vi "Kazu_randstim_TMStrigger and cleaned_ver2.vi"() -> ()   [LabVIEW 2011]
uses:
  <vilib>/Analysis/NI_AALBase.lvlib
  <vilib>/DAQmx/create/channels.llb/DAQmx Create Channel (DO-Digital Output).vi
  <vilib>/DAQmx/write.llb/DAQmx Write (Digital Bool 1Line 1Point).vi
  <vilib>/Utility/file.llb/Read Delimited Spreadsheet (I64).vi
  <vilib>/Platform/TimedLoop/XDataNode/wakeup.ctl
  <vilib>/Platform/TimedLoop/XDataNode/XDNodeRunTimeDep.lvlib
  <vilib>/Platform/TimedLoop/XDataNode/nitl_modes.ctl
  <vilib>/Platform/TimedLoop/XDataNode/timing_clust.ctl
  <vilib>/platform/TimedLoop/XDataNode/XDataNode.xnode
  <vilib>/Analysis/baseanly.llb/A x Vector.vi
  <vilib>/Utility/file.llb/Write Delimited Spreadsheet (DBL).vi
  <vilib>/Platform/TimedLoop/scheduler/LVUserAPI/_suppVIs/Create_1kHz_TSource.vi
panel:
  in  "train length (ms)":i64=500
  out "TMS trigger send":bool
  in  "H duration (ms)":i32=10 min=5 max=15
  in  "DO duration (ms)":i32=500
  in  "nominal freq (Hz)":i32=40
  in  "percent for random":dbl=20.0
  out "Digital Waveform Graph":digitalwaveform(graph)={"t0"=timestamp(0 s since 1904-01-01), "dt"=0.001, "Y"={"transitions"=[], "data"=[[1], [1], [1], [1], [1], [1], [1], [1], [1], [1], [0], [0], [0], [0], [0], [0], [0], [0], [0], [0], [0], [0], [0], [0], [0], [0], [1], [1], [1], [1], [1], [1], [1], [1], [1], [1], [0], [0], [0], [0], [0], [0], [0], [0], [0], [0], [0], [0], [0], [0], [0], [1], [1], [1], [1], [1], [1], [1], [1], [1], [1], [0], [0], [0], [0], [0], [0], [0], [0], [0], [0], [0], [0], [0], [0], [1], [1], [1], [1], [1], [1], [1], [1], [1], [1], [0], [0], [0], [0], [0], [0], [0], [0], [0], [0], [0], [0], [0], [0], [0], [1], [1], [1], [1], [1], [1], [1], [1], [1], [1], [0], [0], [0], [0], [0], [0], [0], [0], [0], [0], [0], [0], [0], [0], [0], [0], [0], [0], [0], [0], [0], [0], [0], [0], [0], [0], [0], [0], [0], [0], [0], [0], [0], [0], [0], [0], [0], [0], [0], [0], [0], [0], [0], [0], [0], [0], [0], [0], [0], [0], [0], [0], [0], [0], [0], [0], [0], [0], [0], [0], [0], [0], [0], [0], [0], [0], [0], [0], [0], [0], [0], [0], [0], [0], [0], [0], [0], [0], [0], [0], [0], [0], [0], [0], [0], [0], [0], [0], [0], [0], [0], [0], [0], [0], [0], [0], [0], [0], [0], [0], [0], [0], [0], [0], [0], [0], [0], [0], [0], [0], [0], [0], [0], [0], [0], [0], [0], [0], [0], [0], [0], [0], [0], [0], [0], [0], [0], [0], [0], [0], [0], [0], [0], [0], [0], [0], [0], [0], [0], [0], [0], [0], [0], [0], [0], [0], [0], [0], [0], [0], [0], [0], [0], [0], [0], [0], [0], [0], [0], [0], [0], [0], [0], [0], [0], [0], [0], [0], [0], [0], [0], [0], [0], [0], [0], [0], [0], [0], [0], [0], [0], [0], [0], [0], [0], [0], [0], [0], [0], [0], [0], [0], [0], [0], [0], [0], [0], [0], [0], [0], [0], [0], [0], [0], [0], [0], [0], [0], [0], [0], [0], [0], [0], [0], [0], [0], [0], [0], [0], [0], [0], [0], [0], [0], [0], [0], [0], [0], [0], [0], [0], [0], [0], [0], [0], [0], [0], [0], [0], [0], [0], [0], [0], [0], [0], [0], [0], [0], [0], [0], [0], [0], [0], [0], [0], [0], [0], [0], [0], [0], [0], [0], [0], [0], [0], [0], [0], [0], [0], [0], [0], [0], [0], [0], [0], [0], [0], [0], [0], [0], [0], [0], [0], [0], [0], [0], [0], [0], [0], [0], [0], [0], [0], [0], [0], [0], [0], [0], [0], [0], [0], [0], [0], [0], [0], [0], [0], [0], [0], [0], [0], [0], [0], [0], [0], [0], [0], [0], [0], [0], [0], [0], [0], [0], [0], [0], [0], [0], [0], [0], [0], [0], [0], [0], [0], [0], [0], [0], [0], [0], [0], [0], [0], [0], [0], [0], [0], [0], [0], [0], [0], [0], [0], [0], [0], [0], [0], [0], [0], [0], [0], [0], [0], [0], [0], [0], [0], [0], [0], [0], [0], [0], [0], [0], [0], [0], [0], [0], [0], [0], [0], [0], [0], [0], [0], [0], [0], [0], [0], [0]]}}
  in  "Trial No":u16(ring)=1 items=["N/A", "Trial 1", "Trial 2", "Trial 3", "Trial 4", "Trial 5", "Trial 6", "Trial 7", "Trial 8", "Trial 9", "Trial 10", "Trial 11", "Trial 12", "Trial 13", "Trial 14", "Trial 15", "Trial 16", "Trial 17", "Trial 18", "Trial 19", "Trial 20", "Trial 21", "Trial 22", "Trial 23", "Trial 24", "Trial 25", "Trial 26", "Trial 27", "Trial 28", "Trial 29", "Trial 30", "Trial 31", "Trial 32", "Trial 33", "Trial 34", "Trial 35", "Trial 36", "Trial 37", "Trial 38", "Trial 39", "Trial 40", "Trial 41", "Trial 42", "Trial 43", "Trial 44", "Trial 45", "Trial 46", "Trial 47", "Trial 48", "Trial 49", "Trial 50", "Trial 51", "Trial 52", "Trial 53", "Trial 54", "Trial 55", "Trial 56", "Trial 57", "Trial 58", "Trial 59", "Trial 60", "Trial 61", "Trial 62", "Trial 63", "Trial 64", "Trial 65", "Trial 66", "Trial 67", "Trial 68", "Trial 69", "Trial 70", "Trial 71", "Trial 72", "Trial 73", "Trial 74", "Trial 75", "Trial 76", "Trial 77", "Trial 78", "Trial 79", "Trial 80", "Trial 81", "Trial 82", "Trial 83", "Trial 84", "Trial 85", "Trial 86", "Trial 87", "Trial 88", "Trial 89", "Trial 90", "Trial 91", "Trial 92", "Trial 93", "Trial 94", "Trial 95", "Trial 96", "Trial 97", "Trial 98", "Trial 99", "Trial 100", "Trial 101", "Trial 102", "Trial 103", "Trial 104", "Trial 105", "Trial 106", "Trial 107", "Trial 108", "Trial 109", "Trial 110", "Trial 111", "Trial 112", "Trial 113", "Trial 114", "Trial 115", "Trial 116", "Trial 117", "Trial 118", "Trial 119", "Trial 120", "Trial 121", "Trial 122", "Trial 123", "Trial 124", "Trial 125", "Trial 126", "Trial 127", "Trial 128", "Trial 129", "Trial 130", "Trial 131", "Trial 132", "Trial 133", "Trial 134", "Trial 135", "Trial 136", "Trial 137", "Trial 138", "Trial 139", "Trial 140", "Trial 141", "Trial 142", "Trial 143", "Trial 144", "Trial 145", "Trial 146", "Trial 147", "Trial 148", "Trial 149", "Trial 150", "Trial 151", "Trial 152", "Trial 153", "Trial 154", "Trial 155", "Trial 156", "Trial 157", "Trial 158", "Trial 159", "Trial 160", "Trial 161", "Trial 162", "Trial 163", "Trial 164", "Trial 165", "Trial 166", "Trial 167", "Trial 168", "Trial 169", "Trial 170", "Trial 171", "Trial 172", "Trial 173", "Trial 174", "Trial 175", "Trial 176", "Trial 177", "Trial 178", "Trial 179", "Trial 180", "Trial 181", "Trial 182", "Trial 183", "Trial 184", "Trial 185", "Trial 186", "Trial 187", "Trial 188", "Trial 189", "Trial 190"]
  out "start":bool
  in  "RECORD":bool
  in  "BNC port for EMG":tag="Dev1/port0/line4" caption="BNC port for EMG and EMG"
  out "sucsess":bool
  out "TMS type":i64=3
  in  "sequence file path_TMS Order":path=path "C:/Users/marco2013/Documents/Kazu/EEG-TMS/rand_stim_study/rand_stim_taskorder/sub9/randStim_TMSOrder_sub9.txt"
  out "x-y":dbl=10.0
  out "checkTime":dbl=16261.0
  in  "MVC clear":bool
  out "MVC value":dbl=23.092750263611816
  in  "MVC recording":bool
  in  "total time":u32=9000
  out "timer":u32=16261
  out "end":bool
  out "go":bool
  out "ready":bool
  out "cue":bool
  out "%MVC":dbl(slide)=-0.42778761105628194 scale=0.0..60.0
  in  "BNC port for TMS":tag="Dev1/port0/line1"
  out "condtion":i64=1
  in  "sequence file path_TASK Order":path=path "C:/Users/marco2013/Documents/Kazu/EEG-TMS/rand_stim_study/rand_stim_taskorder/sub9/randStim_TaskOrder_sub9.txt"
  out "Force":dbl=-0.09878792467989823
  in  "Block":u16(ring)=1 items=["N/A", "Block 1", "Block 2", "Block 3", ""]
  in  "string":string="C:\\Users\\marco2013\\Documents\\Kazu\\EEG-TMS\\rand_stim_study\\"
  out "path":path=path "C:/Users/marco2013/Documents/Kazu/EEG-TMS/rand_stim_study/FT0101190.txt"
  in  "Subject":u16(ring)=9 items=["N/A", "Sub 1", "Sub 2", "Sub 3", "Sub 4", "Sub 5", "Sub 6", "Sub 7", "Sub 8", "Sub 9", "Sub 10", "Sub 11", "Sub 12", "Sub 13", "Sub 14", "Sub 15"]
  in  "number of samples":i32=10
  in  "device name":tag="Dev1"
  in  "Sampling rate":dbl=1000.0
  out "Array":dbl[][](array[numeric])=[[0.0, 0.0, 0.0, 0.0, 0.0, 0.0], [0.0, 0.0, 0.0, 0.0, 0.0, 0.0], [0.0, 0.0, 0.0, 0.0, 0.0, 0.0], [0.0, 0.0, 0.0, 0.0, 0.0, 0.0], [0.2289245236771016, -0.066272275562497, 0.09878792467989823, 0.001145934848439327, -0.0024626830830202645, -0.003738509500700172]]
  in  "stop":bool=TRUE
  in  "Bias All":bool
  in  "Enable Transducer 2":bool[](array[boolean])=[TRUE, TRUE, TRUE, TRUE, TRUE]
  in  "Calibration Files":path[](array[path])=[path "C:/Users/marco2013/Documents/Kazu/bigbox/FT6124.cal", path "C:/Users/marco2013/Documents/Kazu/bigbox/FT6561.cal", path "C:/Users/marco2013/Documents/Kazu/bigbox/FT4554.cal", path "C:/Users/marco2013/Documents/Kazu/bigbox/FT16536.cal", path "C:/Users/marco2013/Documents/Kazu/bigbox/FT14450.cal"]
  # "1: catch\n2: 20Hz stim\n3: 50Hz stim"
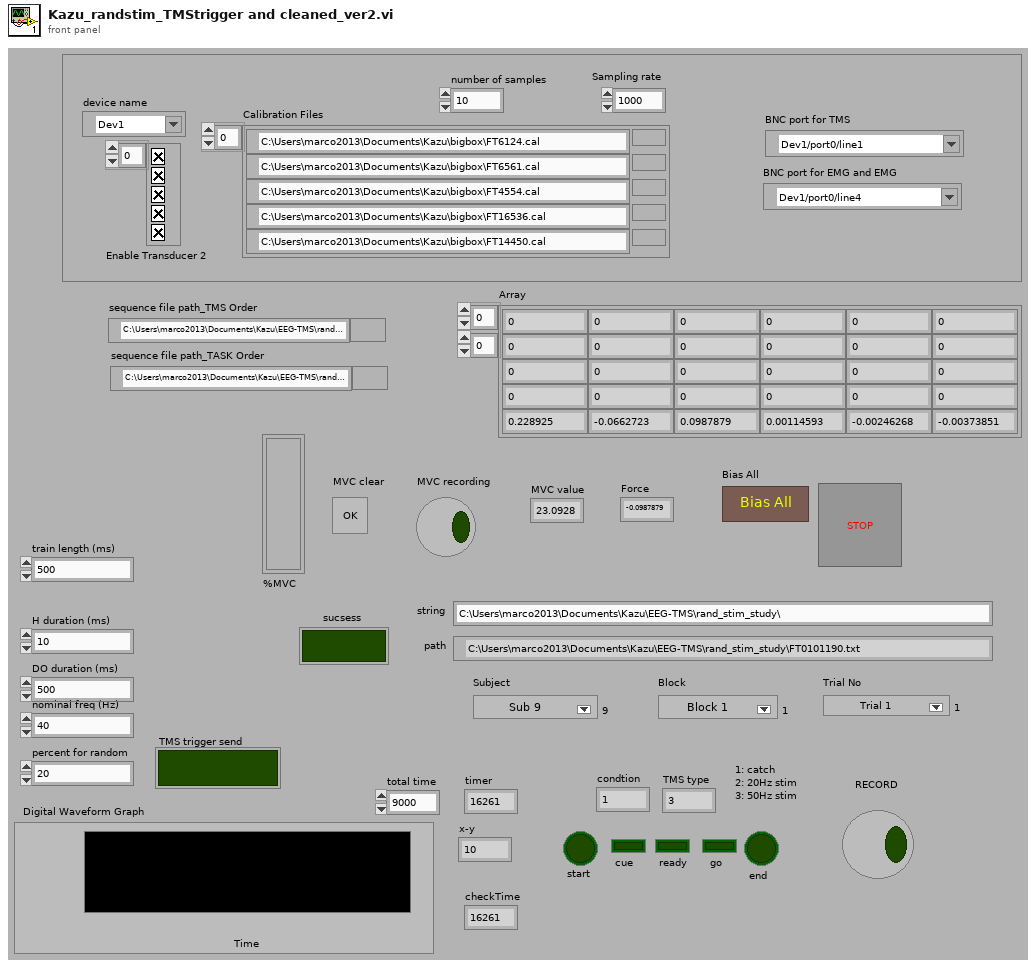
[diagram p1: front panel]
types:
  T1 = enum16{"open", "replace", "create", "open or create", "replace or create", "replace or create with confirmation"}
  T2 = enum16{"open", "open or create", "create or replace", "create", "open (read-only)"}
  T3 = typedef "XDNodeRunTimeDep.lvlib/timing_clust.ctl" = cluster{"Expected End [f-1]":u64, "Actual End [f-1]":u64, "Finished Late? [f-1]":bool, "Expected End [i-1]":u64, "Actual End [i-1]":u64, "Finished Late? [i-1]":bool, "Expected Start [i]":u64, "Actual Start [i]":u64, "Expected Start [f]":u64, "Actual Start [f]":u64, "Source Name":string, "Structure Name":string, "Period":i64, "Deadline":i64, "Offset":i64, "Start":i64, "Priority":i32, "Timeout":i32, "Mode":T4, "Wakeup Reason":T5, "Error":errorcluster, "Source Type":string, "Secondary Source Type":string, "Global End Time":u64, "Global Start Time":u64, "Frame Duration":u64, "Iteration Duration":u64, "Assigned CPU":i32, "I/O Scan Engine Mode":u32}
  T4 = typedef "XDNodeRunTimeDep.lvlib/nitl_modes.ctl" = enum32{"No Change", "Process missed periods, maintain original phase", "Discard missed periods, maintain original phase", "Process missed periods, ignore original phase", "Discard missed periods, ignore original phase"}
  T5 = typedef "XDNodeRunTimeDep.lvlib/wakeup.ctl" = enum32{"Normal", "Aborted", "Asynchronous wakeup", "Timing source error", "Timed loop error", "Timeout"}
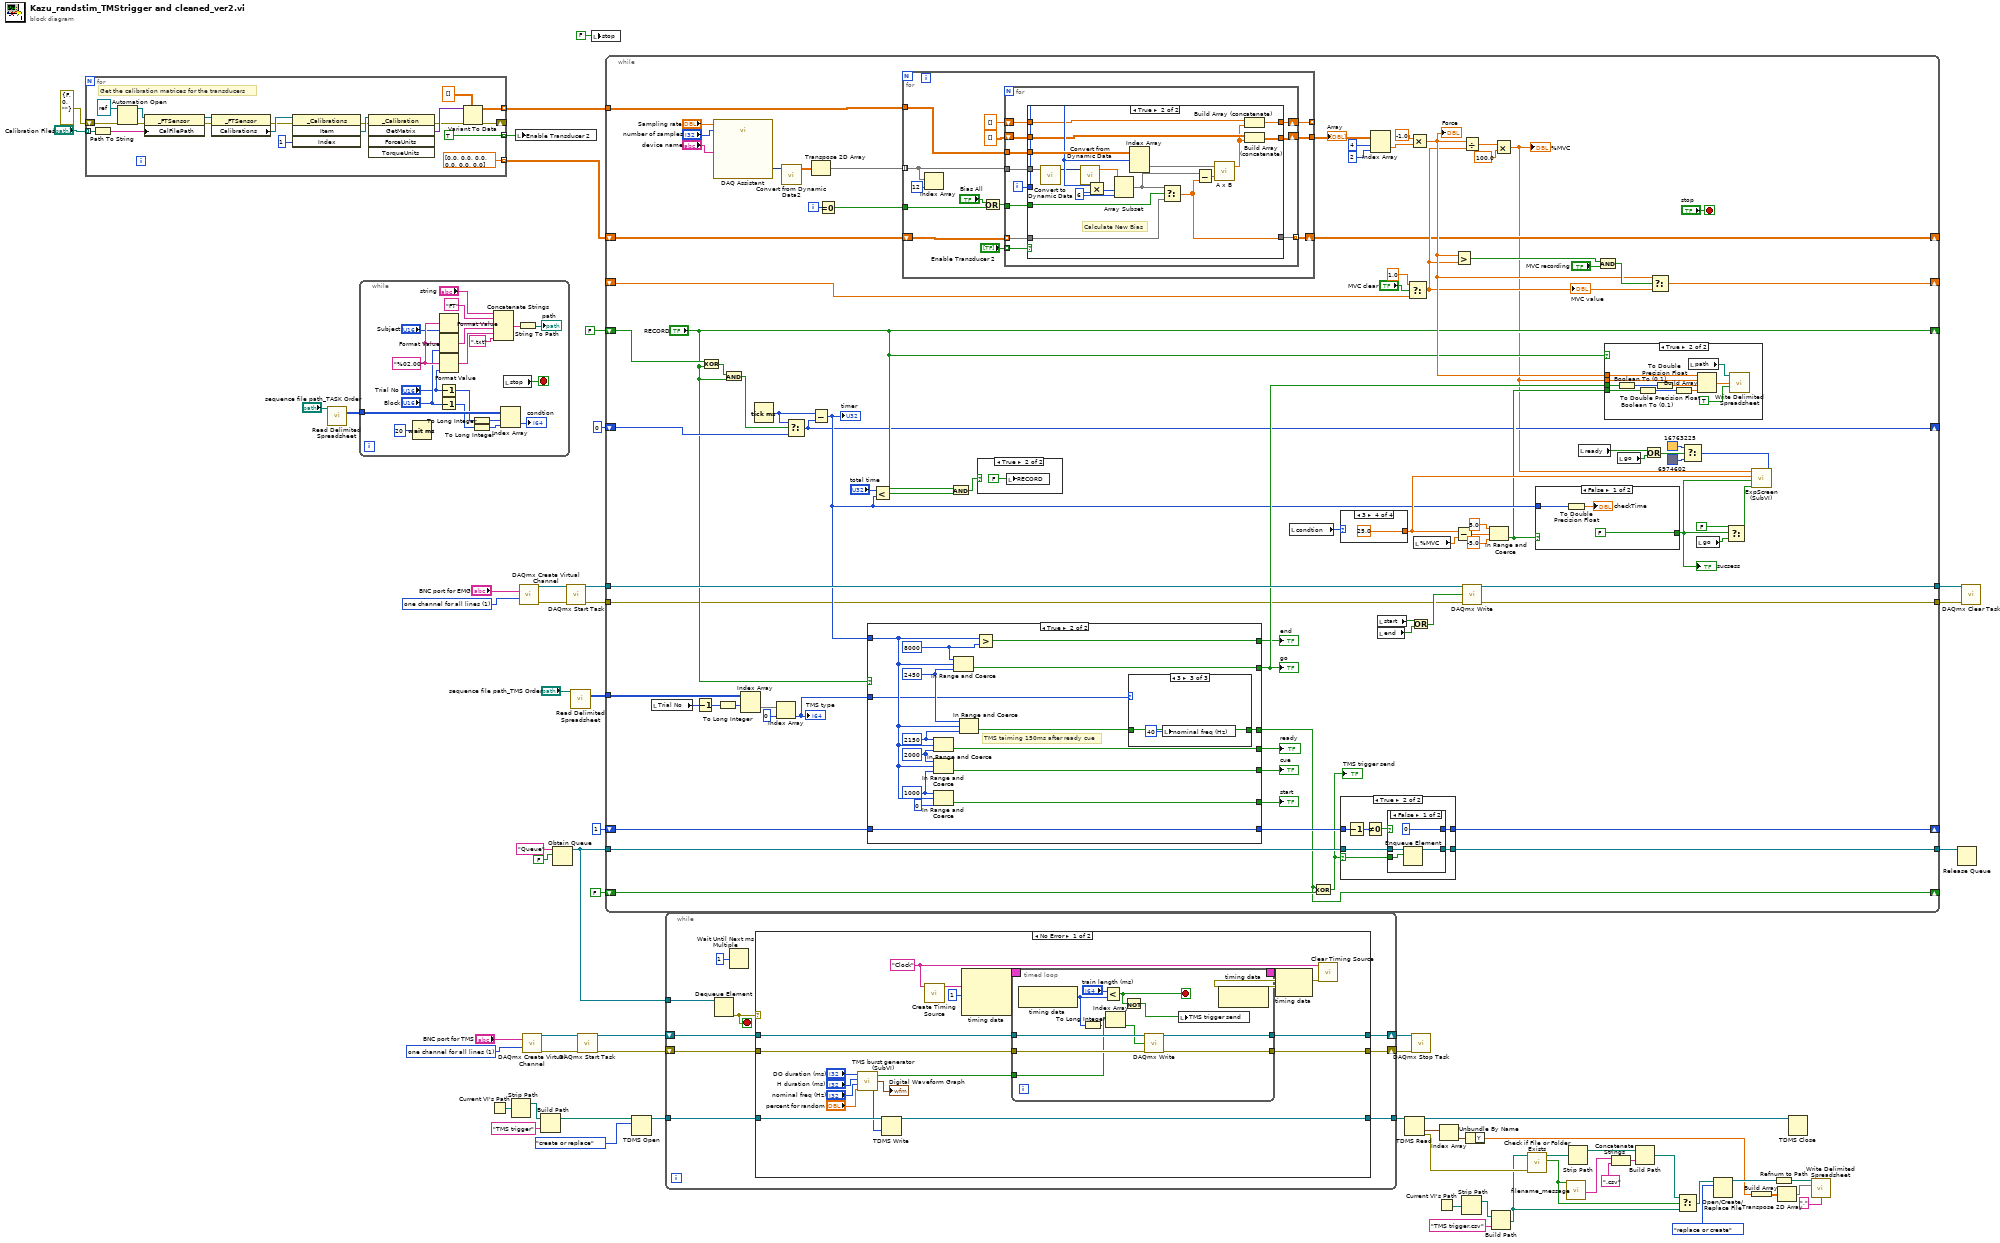
[diagram p0: block diagram]
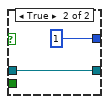
[diagram p4: hidden frame]
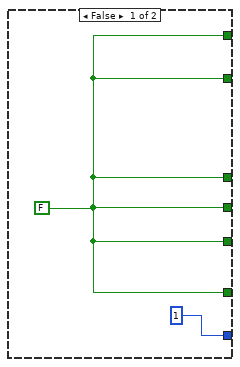
[diagram p6: hidden frame]
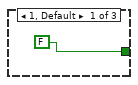
[diagram p7: hidden frame]
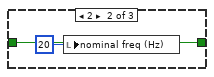
[diagram p8: hidden frame]
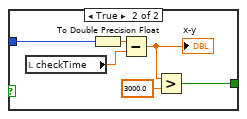
[diagram p9: hidden frame]
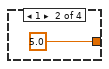
[diagram p11: hidden frame]
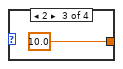
[diagram p12: hidden frame]
diagram:
  w51 = 1 items=["one channel for each line", "one channel for all lines"] ("line grouping")
  w55 = 1 items=["one channel for each line", "one channel for all lines"] ("line grouping")
  n1 = for {
    tunnel: "Calibration Files" -> [w81] mode=indexing
    shift-right: [w72] -> _
    shift-left: errorcluster {"status"=FALSE, "code"=0, "source"=""} ("error out") -> [w69]
    tunnel: [sgl[] [0.0, 0.0, 0.0, 0.0, 0.0, 0.0]] -> w60 mode=indexing
    tunnel: [TRUE] -> w62 mode=indexing
    tunnel: [w65] -> w61 mode=indexing
    # "Get the calibration matrices for the transducers"
    n2 = Path To String(path=w81) -> (string=w80:string)
    n3 = Automation Open(error in (no error)=w69, Automation Refnum=refnum<k7> refnum ("ATIDAQFT._FTSensor")) -> (Automation Refnum=w70:refnum<k7>, error out=w68:errorcluster)  [unwired: 1 in, 1 out]
    n4 = property on="Property Node" class="_FTSensor"(reference=w70, error in=w68, "CalFilePath"=w80) -> (reference out=w82:refnum<k7>, error out=w76:errorcluster)
    n5 = property class="_FTSensor"(reference=w82, error in=w76) -> (error out=w75:errorcluster, "Calibrations"=w84:refnum<k7>)  [unwired: 1 out]
    n6 = invoke class="_Calibrations" method="Item"(reference=w84, error in=w75, "Index"=1) -> (error out=w74:errorcluster, "Item"=w79:refnum<k7>)  [unwired: 1 in, 2 out]
    n7 = invoke class="_Calibration" method="GetMatrix"(reference=w79, error in=w74) -> (error out=w73:errorcluster, "GetMatrix"=w78:variant)  [unwired: 3 in, 3 out]
    n8 = Variant To Data(error in=w73, type=sgl[][] [], Variant=w78) -> (data=w65:sgl[][], error out=w72:errorcluster)
  }
  n9 = call-poly <vilib>:"Read Delimited Spreadsheet.vi"("file path (dialog if empty)"="sequence file path_TASK Order") -> ("all rows"=w56:i64[][])  [unwired: 9 in, 5 out]
  n10 = while {
    tunnel: w56 -> [w92]
    stop <- w104 stop-if-true
    w103 = "%02.00" ("string (\"\")")
    n11 = Wait (ms)(milliseconds to wait=u32 20) -> ()  [unwired: 1 out]
    n12 = Format Value(format string=w103, value (0)="Subject") -> (output string=w96:string)  [unwired: 1 out]
    n13 = Format Value(format string=w103, value (0)="Block") -> (output string=w102:string)  [unwired: 1 out]
    n14 = Format Value(format string=w103, value (0)="Trial No") -> (output string=w101:string)  [unwired: 1 out]
    n15 = Decrement(x="Trial No") -> (x-1=w90:u16)
    n16 = Decrement(x="Block") -> (x-1=w89:u16)
    n17 = To Long Integer(number=w90) -> (32bit integer=w86:i32)
    n18 = To Long Integer(number=w89) -> (32bit integer=w85:i32)
    n19 = Concatenate Strings("string", "FT", w96, w102, w101, ".txt") -> (w94:string)
    n20 = Index Array(array=w92, index (row)=w86, index (col)=w85) -> (element=→"condtion":i64)
    n21 = local read "stop"() -> (w104:bool)
    n22 = String To Path(string=w94) -> (path=→"path":path)
  }
  n23 = Current VI's Path() -> (path=w28:path)
  n24 = Strip Path(path=w28) -> (stripped path=w27:path)  [unwired: 1 out]
  n25 = local write "Enable Transducer 2"(w62) -> ()
  n26 = call-poly <vilib>:"DAQmx Create Virtual Channel.vi"("lines"="BNC port for EMG", "line grouping"=w51) -> ("task out"=w48:refnum<k21>, "error out"=w49:errorcluster)  [unwired: 3 in, 9 out]
  n27 = call-poly <vilib>:"DAQmx Create Virtual Channel.vi"("lines"="BNC port for TMS", "line grouping"=w55) -> ("task out"=w38:refnum<k21>, "error out"=w37:errorcluster)  [unwired: 3 in, 9 out]
  n28 = Build Path(base path=w27, name or relative path="TMS trigger") -> (appended path=w26:path)
  n29 = Obtain Queue(name (unnamed)="Queue", element data type=FALSE) -> (queue out=w33:refnum<queue>)  [unwired: 3 in, 2 out]
  n30 = call <vilib>:"DAQmx Start Task.vi"("task/channels in"=w48, "error in"=w49) -> ("task out"=w46:refnum<k21>, "error out"=w44:errorcluster)  [unwired: 12 out]
  n31 = call-poly <vilib>:"Read Delimited Spreadsheet.vi"("file path (dialog if empty)"="sequence file path_TMS Order") -> ("all rows"=w52:i64[][])  [unwired: 9 in, 5 out]
  n32 = call <vilib>:"DAQmx Start Task.vi"("task/channels in"=w38, "error in"=w37) -> ("task out"=w42:refnum<k21>, "error out"=w40:errorcluster)  [unwired: 12 in]
  n33 = local write "stop"(FALSE ("stop")) -> ()
  n34 = while {
    tunnel: w61 -> [w187]
    shift-right: [w159] -> _
    shift-left: w60 -> [w188]
    shift-right: ["RECORD"] -> _
    shift-left: FALSE -> [w176]
    shift-right: [w120] -> _
    shift-left: u32 0 ("millisecond timer value") -> [w136]
    shift-right: [w164] -> _
    shift-left: _ -> [w161]
    tunnel: w52 -> [w151]
    tunnel: [w149] -> w47
    tunnel: w46 -> [w148]
    tunnel: w44 -> [w116]
    tunnel: [w115] -> w43
    tunnel: w33 -> [w111]
    shift-right: [w108] -> _
    shift-left: FALSE ("RECORD") -> [w114]
    tunnel: [w109] -> w34
    shift-right: [w110] -> _
    shift-left: 1 -> [w113]
    i -> [w181]
    stop <- "stop" stop-if-true
    n35 = local read "Trial No"() -> (w119:u16)
    n36 = Decrement(x=w119) -> (x-1=w118:u16)
    n37 = Exclusive Or(1:"RECORD", 2:w176) -> (0:w135:bool)
    n38 = call "DAQ Assistant"("rate"="Sampling rate", "number of samples"="number of samples", "device name"="device name") -> ("data"=w184:dynamicdata)  [unwired: 3 in, 13 out]
    n39 = To Long Integer(number=w118) -> (32bit integer=w117:i32)
    n40 = And(x=w135, y="RECORD") -> (x .and. y?=w138:bool)
    n41 = Index Array(array=w151, index (row)=w117) -> (element=w152:i64[])  [unwired: 1 in]
    n42 = Tick Count (ms)() -> (millisecond timer value=w137:u32)
    n43 = Index Array(array=w152, index=0) -> (element=w150:i64)
    "TMS type" <- w150
    n44 = call "Convert from Dynamic Data2"("Dynamic Data Type"=w184) -> ("Array"=w183:dbl[][])  [unwired: 3 out]
    n45 = Select(t=w137, s=w138, f=w136) -> (s? t:f=w120:u32)
    n46 = Transpose 2D Array(2D array=w183) -> (transposed array=w182:dbl[][])
    n47 = Subtract(x=w137, y=w120) -> (x-y=w130:u32)
    "timer" <- w130
    n48 = Equal To 0?(x=w181) -> (x = 0?=w185:bool)
    n49 = case shown="True" "RECORD" {
      tunnel: [w206 w222] -> w139
      tunnel: [w206 w221] -> w145
      tunnel: [w206 w220] -> w141
      tunnel: [w206 w219] -> w140
      tunnel: [w206 w218] -> w146
      tunnel: w130 -> [_ w217]
      tunnel: [w206 w208] -> w108
      tunnel: w150 -> [_ w210]
      tunnel: [1 w216] -> w112
      tunnel: w113 -> [_ w216]
      frame False {
        w206 = FALSE ("RECORD")
      }
      frame True {
        w211 = u32 2450 ("upper limit")
        w212 = u32 8000 ("upper limit")
        w207 = u32 2150 ("upper limit")
        w213 = u32 2000 ("upper limit")
        w214 = u32 1000 ("upper limit")
        # "TMS taiming 150ms after ready cue"
        n50 = In Range and Coerce(upper limit=w207, x=w217, lower limit=w213) -> (In Range?=w219:bool)  [unwired: 1 out]
        n51 = In Range and Coerce(upper limit=w213, x=w217, lower limit=w214) -> (In Range?=w221:bool)  [unwired: 1 out]
        n52 = In Range and Coerce(upper limit=w214, x=w217, lower limit=u32 0) -> (In Range?=w222:bool)  [unwired: 1 out]
        n53 = In Range and Coerce(upper limit=w212, x=w217, lower limit=w211) -> (In Range?=w218:bool)  [unwired: 1 out]
        n54 = In Range and Coerce(upper limit=w211, x=w217, lower limit=w207) -> (In Range?=w209:bool)  [unwired: 1 out]
        n55 = Greater?(x=w217, y=w212) -> (0:w220:bool)
        n56 = case shown="3" w210 {
          tunnel: w209 -> [_ w224 w226]
          tunnel: [FALSE w224 w226] -> w208
          frame 1, Default {
          }
          frame 2 {
            n57 = local write "nominal freq (Hz)"(20 ("x")) -> ()
          }
          frame 3 {
            n58 = local write "nominal freq (Hz)"(40 ("x")) -> ()
          }
        }
      }
    }
    "ready" <- w140
    "cue" <- w145
    "go" <- w146
    "end" <- w141
    "start" <- w139
    n59 = Less?(x="total time", y=w130) -> (x < y?=w170:bool)
    n60 = for {
      tunnel: w182 -> [w252] mode=indexing
      tunnel: w187 -> [w263]
      shift-right: [w261] -> w159
      shift-left: w188 -> [w255]
      tunnel: w185 -> [w256]
      tunnel: [w254] -> w169
      tunnel: [w251] -> _ mode=indexing
      n61 = Index Array(array=w252, index=12) -> ()  [unwired: 1 out]
      n62 = Or(x="Bias All", y=w256) -> (x .or. y?=w257:bool)
      n63 = for {
        tunnel: w263 -> [w271]
        tunnel: w252 -> [w274]
        tunnel: w255 -> [w273] mode=indexing
        tunnel: [w272] -> w261 mode=indexing
        shift-right: [w264] -> w251
        shift-left: dbl[] [] -> [w269]
        tunnel: "Enable Transducer 2" -> [w268] mode=indexing
        shift-right: [w266] -> w254
        shift-left: sgl[][] [] -> [w267]
        tunnel: w257 -> [w265]
        i -> [w270]
        n64 = case shown="True" w268 {
          tunnel: w274 -> [_ w293]
          tunnel: w273 -> [w277 w279]
          tunnel: [w277 w280] -> w272
          tunnel: w271 -> [_ w291]
          tunnel: w270 -> [_ w289]
          tunnel: w269 -> [w276 w285]
          tunnel: [w276 w283] -> w264
          tunnel: w267 -> [w275 w288]
          tunnel: [w275 w287] -> w266
          tunnel: w265 -> [_ w281]
          frame False {
          }
          frame True {
            w294 = 6
            # "Calculate New Bias"
            n65 = call "Convert to Dynamic Data"("Array"=w293) -> ("Dynamic Data Type"=w282:dynamicdata)  [unwired: 3 out]
            n66 = call "Convert from Dynamic Data"("Dynamic Data Type"=w282) -> ("Array"=w286:dbl[])  [unwired: 3 out]
            n67 = Multiply(x=w289, y=w294) -> (x*y=w295:i32)
            n68 = Array Subset(array=w286, index=w295, length=w294) -> (w278:dbl[])
            n69 = Index Array(array=w291, index (dim 0)=w289) -> (element=w290:sgl[][])  [unwired: 2 in]
            n70 = Select(t=w278, s=w281, f=w279) -> (s? t:f=w280:dbl[])
            n71 = Subtract(x=w278, y=w280) -> (x-y=w292:dbl[])
            n72 = call-poly <vilib>:"A x B.vi"("Vector"=w292, "A"=w290) -> ("A x Vector"=w284:dbl[])  [unwired: 1 out]
            n73 = Build Array (concatenate)(w285, w284) -> (w283:dbl[])
            n74 = Build Array (concatenate)(w288, w284) -> (w287:dbl[][])
          }
        }
      }
    }
    "Array" <- w169
    n75 = And(x="RECORD", y=w170) -> (x .and. y?=w147:bool)
    n76 = case shown="True" w147 {
      frame False {
      }
      frame True {
        n77 = local write "RECORD"(FALSE ("RECORD")) -> ()
      }
    }
    n78 = local read "condtion"() -> (w158:i64)
    n79 = Exclusive Or(1:w114, 2:w108) -> (0:w107:bool)
    "TMS trigger send" <- w107
    n80 = case shown="3" w158 {
      tunnel: [_ 5.0 10.0 25.0] -> w157
      frame 0, Default {
      }
      frame 1 {
      }
      frame 2 {
      }
      frame 3 {
      }
    }
    n81 = case shown="True" w107 {
      selector: w107 -> [_ w194]
      tunnel: w112 -> [w190 w197]
      tunnel: w111 -> [w189 w193]
      tunnel: [w190 w192] -> w110
      tunnel: [w189 w191] -> w109
      frame False {
      }
      frame True {
        n82 = Decrement(x=w197) -> (x-1=w196:i32)
        n83 = Not Equal To 0?(x=w196) -> (x != 0?=w195:bool)
        n84 = case shown="False" w195 {
          tunnel: [0 1] -> w192
          tunnel: w194 -> [w201 _]
          tunnel: w193 -> [w200 w202]
          tunnel: [w198 w202] -> w191
          frame False {
            n85 = Enqueue Element(queue=w200, element=w201) -> (queue out=w198:refnum<queue>)  [unwired: 2 in, 2 out]
          }
          frame True {
          }
        }
      }
    }
    n86 = Index Array(array=w169, index (row)=4, index (col)=2 ("disabled index (col)")) -> (element=w175:dbl)
    n87 = local read "start"() -> (w144:bool)
    n88 = local read "end"() -> (w143:bool)
    n89 = Select(t=1.0 ("f"), s="MVC clear", f=w161) -> (s? t:f=w160:dbl)
    "MVC value" <- w160
    n90 = Multiply(x=-1.0, y=w175) -> (x*y=w165:dbl)
    "Force" <- w165
    n91 = Or(x=w144, y=w143) -> (x .or. y?=w142:bool)
    n92 = local read "%MVC"() -> (w156:dbl)
    n93 = Greater?(x=w165, y=w160) -> (0:w168:bool)
    n94 = Subtract(x=w157, y=w156) -> (x-y=w124:dbl)
    n95 = Divide(x=w165, y=w160) -> (x/y=w172:dbl)
    n96 = call-poly <vilib>:"DAQmx Write.vi"("task/channels in"=w148, "data"=w142, "error in"=w116) -> ("task out"=w149:refnum<k21>, "error out"=w115:errorcluster)  [unwired: 10 in, 1 out]
    n97 = In Range and Coerce(upper limit=5.0 ("y"), x=w124, lower limit=-5.0 ("y")) -> (In Range?=w122:bool)  [unwired: 1 out]
    n98 = Multiply(x=w172, y=100.0) -> (x*y=w106:dbl)
    "%MVC" <- w106
    n99 = case shown="False" w122 {
      tunnel: w130 -> [w230 w234]
      tunnel: [FALSE ("RECORD") w233] -> w128
      frame False {
        n100 = To Double Precision Float(number=w230) -> (double precision float=→"checkTime":dbl)
      }
      frame True {
        n101 = local read "checkTime"() -> (w235:dbl)
        n102 = To Double Precision Float(number=w234) -> (double precision float=w231:dbl)
        n103 = Subtract(x=w231, y=w235) -> (x-y=w232:dbl)
        "x-y" <- w232
        n104 = Greater?(x=w232, y=3000.0) -> (0:w233:bool)
      }
    }
    "sucsess" <- w128
    n105 = local read "ready"() -> (w154:bool)
    n106 = And(x=w168, y="MVC recording") -> (x .and. y?=w166:bool)
    n107 = case shown="True" "RECORD" {
      tunnel: w146 -> [_ w248]
      tunnel: w165 -> [_ w250]
      tunnel: w106 -> [_ w249]
      tunnel: w122 -> [_ w242]
      frame False {
      }
      frame True {
        n108 = Boolean To (0,1)(Boolean=w248) -> (0, 1=w247:i16)
        n109 = Boolean To (0,1)(Boolean=w242) -> (0, 1=w243:i16)
        n110 = To Double Precision Float(number=w247) -> (double precision float=w241:dbl)
        n111 = To Double Precision Float(number=w243) -> (double precision float=w240:dbl)
        n112 = local read "path"() -> (w245:path)
        n113 = Build Array(w250, w249, w241, w240) -> (w246:dbl[])
        n114 = call-poly <vilib>:"Write Delimited Spreadsheet.vi"("file path (dialog if empty)"=w245, "1D data"=w246, "append to file? (F)"=TRUE) -> ()  [unwired: 11 in, 2 out]
      }
    }
    n115 = local read "go"() -> (w155:bool)
    n116 = Or(x=w154, y=w155) -> (x .or. y?=w131:bool)
    n117 = Select(t=w165, s=w166, f=w160) -> (s? t:f=w164:dbl)
    n118 = Select(t=u32 16763225, s=w131, f=u32 6974602) -> (s? t:f=w105:u32)
    n119 = local read "go"() -> (w126:bool)
    n120 = Select(t=FALSE ("append to file? (F)"), s=w128, f=w126) -> (s? t:f=w127:bool)
    n121 = call "ExpScreen (SubVI).vi"("Color Box"=w105, "go in"=w127, "end in"=w128, "value in"=w157, "%MVC in"=w106) -> ()
  }
  n122 = TDMS Open(10:T2."create or replace" ("operation (0:open)"), 11:w26) -> (3:w30:refnum<k34>)  [unwired: 4 in, 1 out]
  n123 = while {
    shift-right: [w303] -> w41
    shift-left: w42 -> [w304]
    shift-right: [w301] -> w39
    shift-left: w40 -> [w302]
    tunnel: w33 -> [w299]
    tunnel: w30 -> [w297]
    tunnel: [w296] -> w24
    stop <- w298 stop-if-true
    n124 = Dequeue Element(queue=w299) -> (error out=w298:errorcluster)  [unwired: 2 in, 3 out]
    n125 = Wait Until Next ms Multiple(millisecond multiple=u32 1) -> ()  [unwired: 1 out]
    n126 = case shown="No Error" w298 {
      tunnel: w304 -> [w323 w346]
      tunnel: [w322 w346] -> w303
      tunnel: w302 -> [w321 w345]
      tunnel: [w320 w345] -> w301
      tunnel: w297 -> [w307 w344]
      tunnel: [w305 w344] -> w296
      frame No Error {
        w310 = "Clock" ("name (in)")
        n127 = call "TMS burst generator (SubVI).vi"("percent for random"="percent for random", "nominal freq (Hz)"="nominal freq (Hz)", "H duration (ms)"="H duration (ms)", "Total duration (ms)"="DO duration (ms)") -> ("Timing (ms)"=w306:i32[], "digital waveform"=→"Digital Waveform Graph":digitalwaveform, "out"=w316:bool[])
        n128 = TDMS Write(0:w307, 9:w306) -> (4:w305:refnum<k34>)  [unwired: 4 in, 3 out]
        n129 = call-poly <vilib>:"Create Timing Source.vi"("name (in)"=w310) -> ("name (out)"=w312:string)  [unwired: 9 in, 1 out]
        n130 = node-c288(w312, i64 1 ("Period")) -> (w315:T3)  [unwired: 1 in]
        n131 = timed-loop {
          tunnel: w323 -> [w334]
          tunnel: [w333] -> w322
          tunnel: w321 -> [w332]
          tunnel: [w331] -> w320
          timing: w315 -> [_]
          timing-out: [_] -> w314
          tunnel: w316 -> [w330]
          stop <- w327 stop-if-true
          n132 = node-c288() -> (w325:i64)  [unwired: 1 in]
          n133 = To Long Integer(number=w325) -> (32bit integer=w328:i32)
          n134 = Less?(x="train length (ms)", y=w325) -> (x < y?=w327:bool)
          n135 = Index Array(array=w330, index=w328) -> (element=w329:bool)
          n136 = Not(x=w327) -> (.not. x?=w326:bool)
          n137 = call-poly <vilib>:"DAQmx Write.vi"("task/channels in"=w334, "data"=w329, "error in"=w332) -> ("task out"=w333:refnum<k21>, "error out"=w331:errorcluster)  [unwired: 10 in, 1 out]
          n138 = local write "TMS trigger send"(w326) -> ()
          n139 = node-c288() -> ()  [unwired: 1 in, 1 out]
        }
        n140 = node-c288(w314) -> (w311:errorcluster)
        n141 = call <vilib>:"Clear Timing Source.vi"("error in (no error)"=w311, "name"=w310) -> ()  [unwired: 8 in, 2 out]
      }
      frame Error {
      }
    }
  }
  n142 = TDMS Read(0:w24) -> (4:w23:refnum<k34>, 10:w22:waveform(dbl)[], 15:w6:errorcluster)  [unwired: 7 in, 3 out]
  n143 = call <vilib>:"DAQmx Stop Task.vi"("task/channels in"=w41, "error in"=w39) -> ()  [unwired: 12 in, 2 out]
  n144 = Current VI's Path() -> (path=w20:path)
  n145 = Index Array(array=w22) -> (element=w21:waveform(dbl))  [unwired: 1 in]
  n146 = Strip Path(path=w20) -> (stripped path=w19:path)  [unwired: 1 out]
  n147 = Unbundle By Name(w21) -> ("Y"=w13:dbl[])
  n148 = Build Path(base path=w19, name or relative path="TMS trigger.csv") -> (appended path=w2:path)
  n149 = call <vilib>:"Check if File or Folder Exists.vi"("error in (no error)"=w6, "path"=w2) -> ("file or folder exists?"=w4:bool, "dup path"=w5:path)  [unwired: 7 in, 1 out]
  n150 = call "filename_message.vi"("Enable"=w4) -> ("FileName"=w7:string)  [unwired: 16 in, 2 out]
  n151 = Strip Path(path=w5) -> (stripped path=w10:path)  [unwired: 1 out]
  n152 = Concatenate Strings(w7, ".csv" ("string")) -> (w9:string)
  n153 = Build Path(base path=w10, name or relative path=w9) -> (appended path=w3:path)
  n154 = Select(t=w3, s=w4, f=w2) -> (s? t:f=w1:path)
  n155 = Open/Create/Replace File(file path (use dialog)=w1, operation (0:open)=T1."replace or create") -> (refnum out=w15:refnum<file>)  [unwired: 4 in, 2 out]
  n156 = Build Array(w13) -> (w12:dbl[][])
  n157 = Refnum to Path(1:w15) -> (0:w14:path)
  n158 = Transpose 2D Array(2D array=w12) -> (transposed array=w11:dbl[][])
  n159 = TDMS Close(11:w23) -> ()  [unwired: 1 in, 2 out]
  n160 = call-poly <vilib>:"Write Delimited Spreadsheet.vi"("file path (dialog if empty)"=w14, "2D data"=w11, "delimiter (\\t)"="," ("delimiter (\\t)")) -> ()  [unwired: 11 in, 2 out]
  n161 = Release Queue(queue=w34) -> ()  [unwired: 2 in, 3 out]
  n162 = call <vilib>:"DAQmx Clear Task.vi"("task in"=w47, "error in"=w43) -> ()  [unwired: 13 in, 1 out]
